vi "FlatToRichcif_plugincore_GetNamesResponse.vi"(5 "OutputClusterType":T1, 11 "InputCluster":T3) -> (3 "OutputCluster":T1)   [LabVIEW 2021, in "CIFCorePlugin_server.lvlib"]
uses:
  CIFCorePlugin_server.lvlib
  cif_plugincore_GetNamesResponse_Flat.ctl
  cif_common_PluginNames_Flat.ctl
  cif_plugincore_GetNamesResponse.ctl
  cif_common_PluginNames.ctl
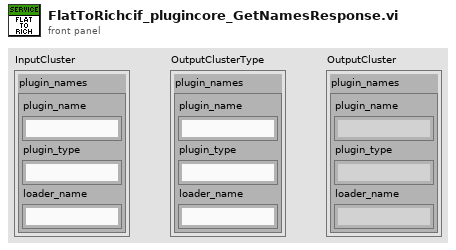
[diagram p1: front panel]
types:
  T1 = typedef "CIFCorePlugin_server.lvlib/cif_plugincore_GetNamesResponse.ctl" = cluster{"plugin_names":T2}
  T2 = typedef "CIFCorePlugin_server.lvlib/cif_common_PluginNames.ctl" = cluster{"plugin_name":string, "plugin_type":string, "loader_name":string}
  T3 = typedef "CIFCorePlugin_server.lvlib/cif_plugincore_GetNamesResponse_Flat.ctl" = cluster{"plugin_names":T4}
  T4 = typedef "CIFCorePlugin_server.lvlib/cif_common_PluginNames_Flat.ctl" = cluster{"plugin_name":string, "plugin_type":string, "loader_name":string}
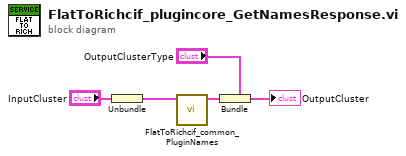
[diagram p0: block diagram]
diagram:
  n1 = Unbundle "Unbundle"("InputCluster") -> ("plugin_names"=w2:T4)
  n2 = call "FlatToRichcif_common_PluginNames.vi"("InputCluster"=w2) -> ("OutputCluster"=w1:T2)  [unwired: 10 in]
  n3 = Bundle "Bundle"(cluster="OutputClusterType", "plugin_names"=w1) -> (→"OutputCluster":T1)
